vi "Append Text to Word Bookmark.vi"(0 "report in":refnum<class "NI_report.lvclass">, 1 "bookmark (word)":string, 7 "text":string, 11 "error in (no error)":errorcluster) -> (4 "report out":refnum<class "NI_report.lvclass">, 15 "error out":errorcluster)   [LabVIEW 2018, in "WordReportGeneration.lvlib" / "Word_Report.lvclass"]
uses:
  Word_Report.lvclass
  <vilib>/Utility/NIReport.llb/NI_report.lvclass
  <vilib>/Utility/NIReport.llb/Append Report Text (str wrap).vi
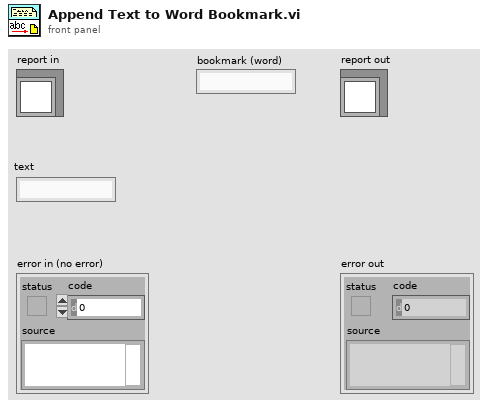
[diagram p1: front panel]
types:
  T1 = cluster{"position (excel)":cluster{"row":i32, "column":i32}, "name (excel)":string, "bookmark (word)":string}
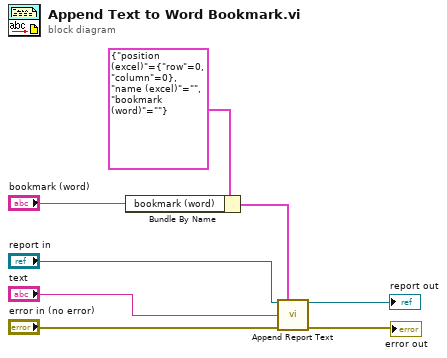
[diagram p0: block diagram]
diagram:
  n1 = Bundle By Name(cluster=T1 {"position (excel)"={"row"=0, "column"=0}, "name (excel)"="", "bookmark (word)"=""} ("MS Office parameters"), "bookmark (word)"="bookmark (word)") -> (w1:T1)
  n2 = call-poly <vilib>:"Append Report Text.vi"("report in"="report in", "MS Office parameters"=w1, "text"="text", "error in (no error)"="error in (no error)") -> ("report out"=→"report out":refnum<class "NI_report.lvclass">, "error out"=→"error out":errorcluster)  [unwired: 8 in, 2 out]
